vi "test.vi"() -> ()   [LabVIEW 2010, in "TIFFManagement.lvlib"]
uses:
  TIFFManagement.lvlib
  classes/Image/Image/target_format_enum.ctl
  VisualCPP/Release/TIFFManagement.dll
panel:
  in  "page":i32
  in  "Tab Control":T1(tab)
  in  "get description button":bool
  out "description":string
  out "Intensity Graph":u32[][](graph)
  in  "get page button":bool
  out "width":i32
  out "height":i32
  out "number of bytes":i32
  in  "single-page target file":path caption="target file"
  in  "write single-page file button":bool
  out "bits per sample":i32
  in  "format?":T2
  in  "description file":path
  in  "multipage target file":path caption="target file"
  in  "write multipage button":bool
  out "number of pages":i32
  in  "get-number-of-pages button":bool
  in  "stop":bool
  in  "input file":path
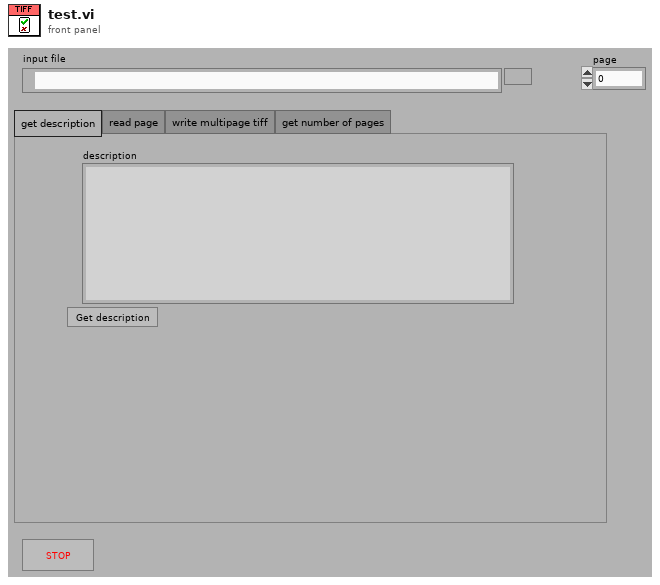
[diagram p1: front panel]
types:
  T1 = enum32{"get description", "read page", "write multipage tiff", "get number of pages"}
  T2 = typedef "target_format_enum.ctl" = enum16{"don't force", "uint8", "uint16", "int16", "uint32", "int32", "single float"}
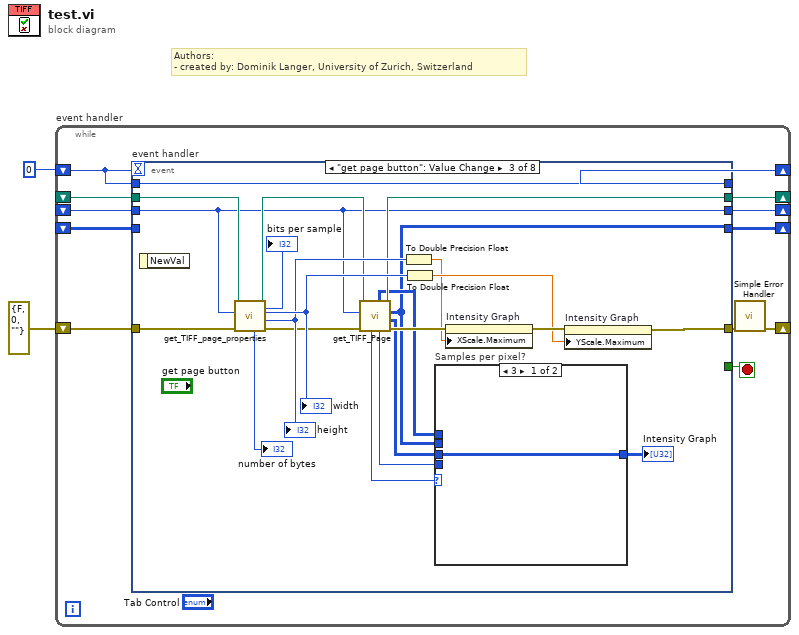
[diagram p0: block diagram]
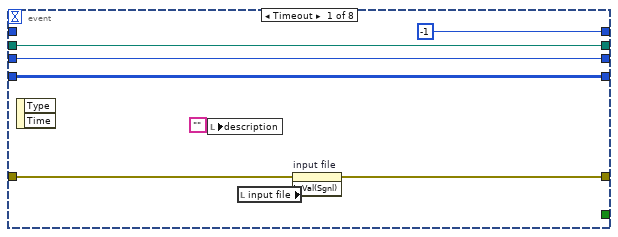
[diagram p2: hidden frame]
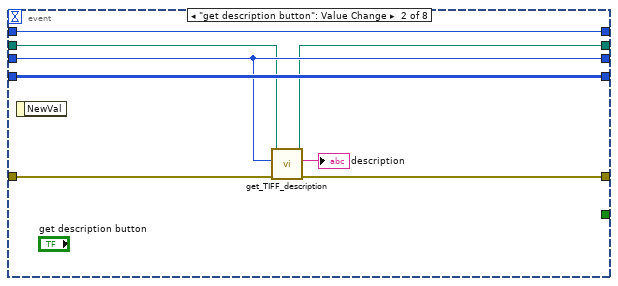
[diagram p3: hidden frame]
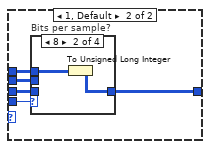
[diagram p4: hidden frame]
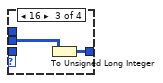
[diagram p6: hidden frame]
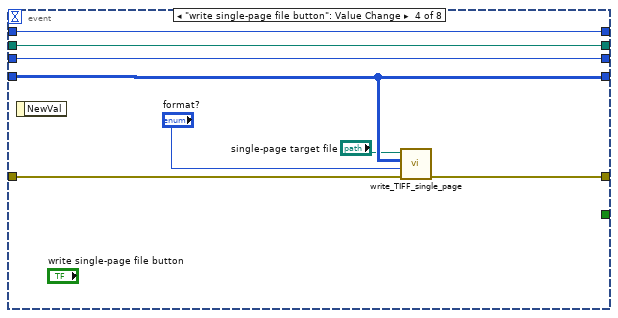
[diagram p8: hidden frame]
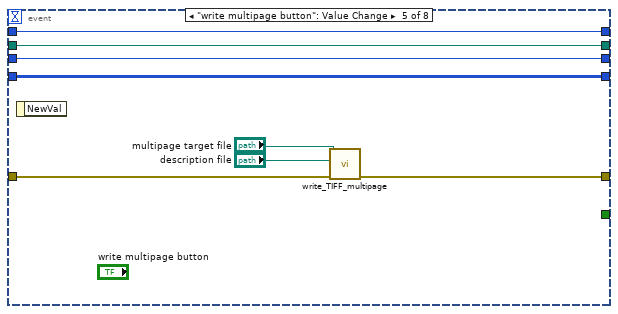
[diagram p9: hidden frame]
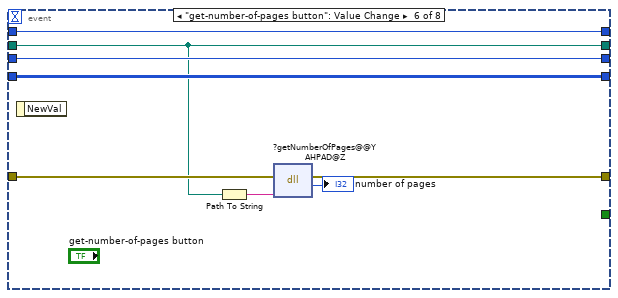
[diagram p10: hidden frame]
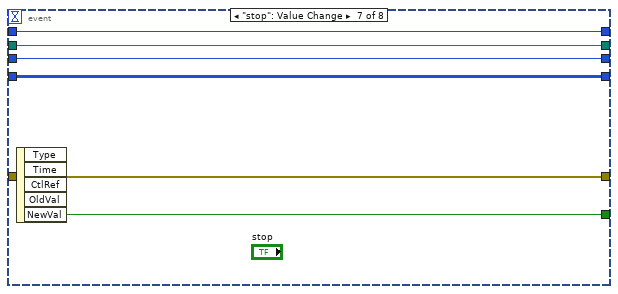
[diagram p11: hidden frame]
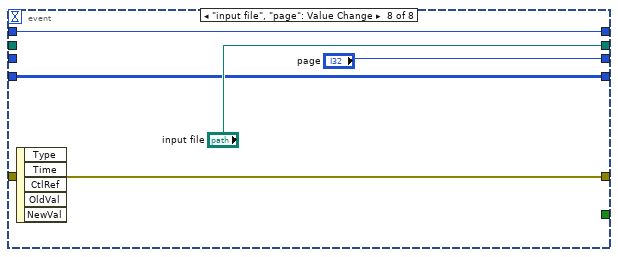
[diagram p12: hidden frame]
diagram:
  # "Authors: \n- created by: Dominik Langer, University of Zurich, Switzerland"
  n1 = while "event handler" {
    shift-right: [w12] -> _
    shift-left: _ -> [w13]
    shift-right: [w8] -> _
    shift-left: errorcluster {"status"=FALSE, "code"=0, "source"=""} ("error out") -> [w11]
    shift-right: [w9] -> _
    shift-left: 0 -> [w10]
    shift-right: [w5] -> _
    shift-left: _ -> [w6]
    shift-right: [w4] -> _
    shift-left: _ -> [w3]
    stop <- w14 stop-if-true
    n2 = event "event handler" shown="[2] \"get page button\": Value Change" {
      selector: _ -> [_ _ _ _ _ _ _ _]
      dyn-events: _ -> [_ _ _ _ _ _ _ _]
      timeout: w10 -> [_ _ _ _ _ _ _ _]
      tunnel: [_ _ _ _ _ _ w93 _] -> w14
      tunnel: w13 -> [w22 w24 w48 w71 w79 w81 w92 _]
      tunnel: [w22 w23 w41 w71 w79 w81 w92 "input file"] -> w12
      tunnel: [w19 w25 w50 w66 w74 w83 w91 w97] -> w7
      tunnel: w11 -> [w20 w28 w49 w67 w75 w84 w91 w97]
      tunnel: [-1 w30 w52 w70 w78 w87 w90 w96] -> w9
      tunnel: w10 -> [_ w30 w52 w70 w78 w87 w90 w96]
      tunnel: w6 -> [w16 w27 w40 w69 w77 w86 w89 _]
      tunnel: [w16 w27 w40 w69 w77 w86 w89 "page"] -> w5
      tunnel: [w15 w29 w35 w68 w76 w85 w88 w94] -> w4
      tunnel: w3 -> [w15 w29 _ w68 w76 w85 w88 w94]
      event Timeout {
        n3 = event-data() -> ()  [unwired: 1 in, 2 out]
        n4 = local write "description"("") -> ()
        n5 = local read "input file"() -> (w18:path)
        n6 = property on="input file" class="Path"(error in=w20, "Val(Sgnl)"=w18) -> (error out=w19:errorcluster)  [unwired: 1 in, 1 out]
      }
      event "get description button": Value Change {
        n7 = event-data() -> ()  [unwired: 1 in, 1 out]
        n8 = call "get_TIFF_description.vi"("error in (no error)"=w28, "page"=w27, "path in"=w24) -> ("error out"=w25:errorcluster, "description"=→"description":string, "path out"=w23:path)  [unwired: 5 in, 1 out]
      }
      event "get page button": Value Change {
        n9 = event-data() -> ()  [unwired: 1 in, 1 out]
        n10 = call "get_TIFF_page_properties.vi"("error in (no error)"=w49, "page"=w40, "path in"=w48) -> ("error out"=w44:errorcluster, "height"=w46:i32, "width"=w47:i32, "path out"=w42:path, "number of bytes"=→"number of bytes":i32, "bits per sample"=→"bits per sample":i32)  [unwired: 2 in, 1 out]
        "height" <- w46
        "width" <- w47
        n11 = call "get_TIFF_Page.vi"("error in (no error)"=w44, "page"=w40, "path in"=w42) -> ("error out"=w43:errorcluster, "data 32bit"=w34:u32[][], "data 16bit"=w35:u16[][], "path out"=w41:path, "bits per sample"=w37:u16, "data 8bit"=w36:u8[][], "samples per pixel"=w32:i32)  [unwired: 2 in]
        n12 = To Double Precision Float(number=w46) -> (double precision float=w38:dbl)
        n13 = To Double Precision Float(number=w47) -> (double precision float=w39:dbl)
        n14 = case "Samples per pixel?" shown="3" w32 {
          tunnel: w37 -> [_ w58]
          tunnel: w36 -> [_ w57]
          tunnel: w35 -> [_ w56]
          tunnel: w34 -> [w53 w55]
          tunnel: [w53 w54] -> w31
          frame 3 {
          }
          frame 1, Default {
            n15 = case "Bits per sample?" shown="8" w58 {
              tunnel: w57 -> [_ w60 _ _]
              tunnel: w56 -> [_ _ w62 _]
              tunnel: w55 -> [_ _ _ w63]
              tunnel: [_ w59 w61 w63] -> w54
              frame 0, Default {
              }
              frame 8 {
                n16 = To Unsigned Long Integer(number=w60) -> (unsigned 32bit integer=w59:u32[][])
              }
              frame 16 {
                n17 = To Unsigned Long Integer(number=w62) -> (unsigned 32bit integer=w61:u32[][])
              }
              frame 32 {
              }
            }
          }
        }
        "Intensity Graph" <- w31
        n18 = property on="Intensity Graph" class="IntGraph (strict)"(error in=w43, "XScale.Maximum"=w38) -> (error out=w51:errorcluster)  [unwired: 1 in, 1 out]
        n19 = property on="Intensity Graph" class="IntGraph (strict)"(error in=w51, "YScale.Maximum"=w39) -> (error out=w50:errorcluster)  [unwired: 1 in, 1 out]
      }
      event "write single-page file button": Value Change {
        n20 = event-data() -> ()  [unwired: 1 in, 1 out]
        n21 = call "write_TIFF_single_page.vi"("error in (no error)"=w67, "force format?"="format?", "data"=w68, "path in"="single-page target file") -> ("error out"=w66:errorcluster)  [unwired: 6 in, 1 out]
      }
      event "write multipage button": Value Change {
        n22 = event-data() -> ()  [unwired: 1 in, 1 out]
        n23 = call "write_TIFF_multipage.vi"("error in (no error)"=w75, "description file"="description file", "path in"="multipage target file") -> ("error out"=w74:errorcluster)  [unwired: 7 in, 1 out]
      }
      event "get-number-of-pages button": Value Change {
        n24 = event-data() -> ()  [unwired: 1 in, 1 out]
        n25 = Path To String(path=w81) -> (string=w82:string)
        n26 = dll-call lib="C:/helioscan/common/libraries/TIFFManagement/VisualCPP/Release/TIFFManagement.dll" fn="?getNumberOfPages@@YAHPAD@Z"(error in=w84, "path"=w82) -> (error out=w83:errorcluster, "return type"=→"number of pages":i32)  [unwired: 3 in, 1 out]
      }
      event "stop": Value Change {
        n27 = event-data() -> ("NewVal"=w93:bool)  [unwired: 1 in, 4 out]
      }
      event "input file", "page": Value Change {
        n28 = event-data() -> ()  [unwired: 1 in, 5 out]
      }
    }
    n29 = call <vilib>:"Simple Error Handler.vi"("error in (no error)"=w7) -> ("error out"=w8:errorcluster)  [unwired: 4 in, 4 out]
  }
